vi "Sort Ascending (single).vi"(8 "error in (no error)":errorcluster, 11 "XY-data":cluster{"X-array":dbl[], "Y-array":dbl[]}) -> (0 "error out":errorcluster, 3 "Sorted XY-data out":cluster{"X-array":dbl[], "Y-array":dbl[]} {"Y-array" format="%.2p"; "X-array" format="%.2p"})   [LabVIEW 2016, in "xy_utilities.lvlib"]
doc: "Sorts the input <b>XY-data</b> according to its x array.\n\nWire data to the data input to determine the polymorphic instance to use or manually select the instance."
uses:
  xy_utilities.lvlib
  <vilib>/Analysis/NI_AALPro.lvlib
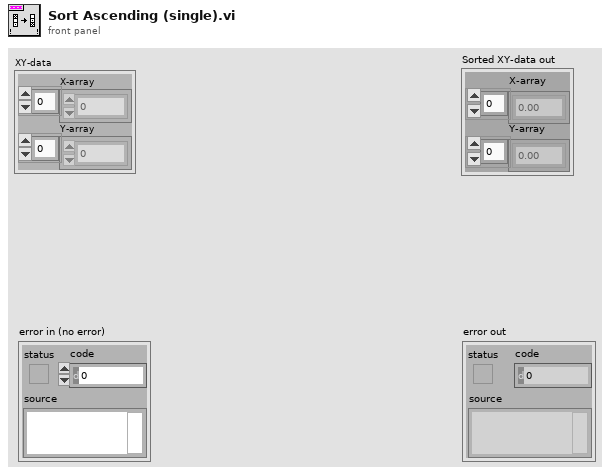
[diagram p1: front panel]
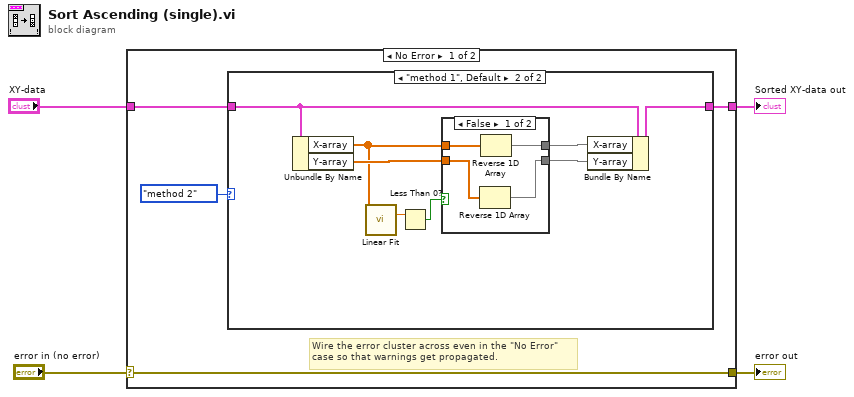
[diagram p0: block diagram]
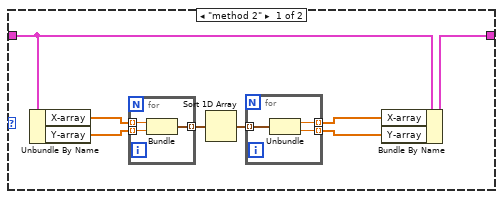
[diagram p2: hidden frame]
diagram:
  n1 = case shown="No Error" "error in (no error)" {
    selector: "error in (no error)" -> [w8 w38]
    tunnel: [w8 w38] -> w3
    tunnel: "XY-data" -> [w7 w37]
    tunnel: [w6 w37] -> w1
    frame No Error {
      # "Wire the error cluster across even in the \"No Error\"\ncase so that warnings get propagated."
      n2 = case shown="\"method 1\", Default" enum16{"method 1", "method 2"}."method 2" {
        tunnel: w7 -> [w10 w30]
        tunnel: [w9 w29] -> w6
        frame "method 2" {
          n3 = Unbundle By Name(w10) -> ("X-array"=w15:dbl[], "Y-array"=w16:dbl[])
          n4 = for {
            tunnel: w15 -> [w19] mode=indexing
            tunnel: w16 -> [w18] mode=indexing
            tunnel: [w17] -> w13 mode=indexing
            n5 = Bundle("x"=w19, "y"=w18) -> (w17:cluster{"x":dbl, "y":dbl})  [unwired: 1 in]
          }
          n6 = Sort 1D Array(array=w13) -> (sorted array=w14:cluster{"x":dbl, "y":dbl}[])
          n7 = for {
            tunnel: w14 -> [w22] mode=indexing
            tunnel: [w21] -> w12 mode=indexing
            tunnel: [w20] -> w11 mode=indexing
            n8 = Unbundle(w22) -> ("x"=w21:dbl, "y"=w20:dbl)
          }
          n9 = Bundle By Name(cluster=w10, "X-array"=w12, "Y-array"=w11) -> (w9:cluster{"X-array":dbl[], "Y-array":dbl[]})
        }
        frame "method 1", Default {
          n10 = Unbundle By Name(w30) -> ("X-array"=w25:dbl[], "Y-array"=w28:dbl[])
          n11 = call <vilib>:"Linear Fit.vi"("Y"=w25) -> ("slope"=w24:dbl)  [unwired: 10 in, 4 out]
          n12 = Less Than 0?(x=w24) -> (x < 0?=w23:bool)
          n13 = case shown="False" w23 {
            tunnel: w25 -> [w34 w36]
            tunnel: w28 -> [w33 w35]
            tunnel: [w32 w35] -> w27
            tunnel: [w31 w36] -> w26
            frame False {
              n14 = Reverse 1D Array(array=w33) -> (reversed array=w32:dbl[])
              n15 = Reverse 1D Array(array=w34) -> (reversed array=w31:dbl[])
            }
            frame True {
            }
          }
          n16 = Bundle By Name(cluster=w30, "X-array"=w26, "Y-array"=w27) -> (w29:cluster{"X-array":dbl[], "Y-array":dbl[]})
        }
      }
    }
    frame Error {
    }
  }
  "error out" <- w3
  "Sorted XY-data out" <- w1
